vi "Uncheck Submenu Items.vi"(7 "Item Tag":string, 8 "error in (no error)":errorcluster, 11 "Menu Ref":refnum<k9>) -> (0 "error out":errorcluster, 3 "Menu Ref out":refnum<k9>)   [LabVIEW 2020, in "VI Properties Editor.lvlib"]
doc: "Unchecks all submenu items of <B>Item Tag</B>."
uses:
  VI Properties Editor.lvlib
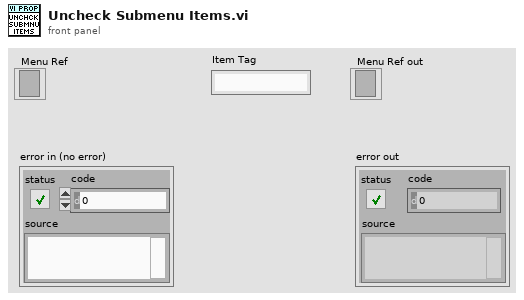
[diagram p1: front panel]
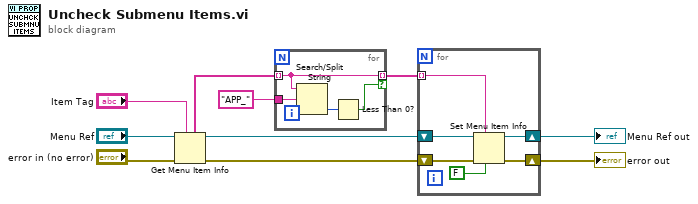
[diagram p0: block diagram]
diagram:
  n1 = Get Menu Item Info(7:"Item Tag", 8:"error in (no error)", 11:"Menu Ref") -> (0:w10:errorcluster, 3:w9:refnum<k9>, 5:w3:string[])  [unwired: 4 out]
  n2 = for {
    tunnel: w3 -> [w13] mode=indexing
    tunnel: "APP_" -> [w14]
    tunnel: [w13] -> w1 mode=indexing if=w11
    n3 = Search/Split String(string=w13, search string/char (-)=w14) -> (offset of match=w12:i32)  [unwired: 1 in, 2 out]
    n4 = Less Than 0?(x=w12) -> (x < 0?=w11:bool)
  }
  n5 = for {
    shift-right: [w18] -> w4
    shift-left: w9 -> [w19]
    shift-right: [w17] -> w5
    shift-left: w10 -> [w16]
    tunnel: w1 -> [w15] mode=indexing
    n6 = Set Menu Item Info(6:FALSE ("checked"), 7:w15, 8:w16, 11:w19) -> (0:w17:errorcluster, 3:w18:refnum<k9>)  [unwired: 3 in]
  }
  "error out" <- w5
  "Menu Ref out" <- w4
